vi "Updater Install Company Logo.vi"(8 "error in (no error)":errorcluster, 10 "Load? (F)":bool, 11 "Path to File":path) -> (0 "error out":errorcluster)   [LabVIEW 2011]
uses:
  <vilib>/picture/picture.llb/imagedata.ctl
panel:
  in  "Image Data":T1={"image type"=0, "image depth"=24, "image"=array[128820 elements], "mask"=[], "colors"=[], "Rectangle"={"left"=0, "top"=0, "right"=380, "bottom"=113}}
  in  "Company Logo":picture
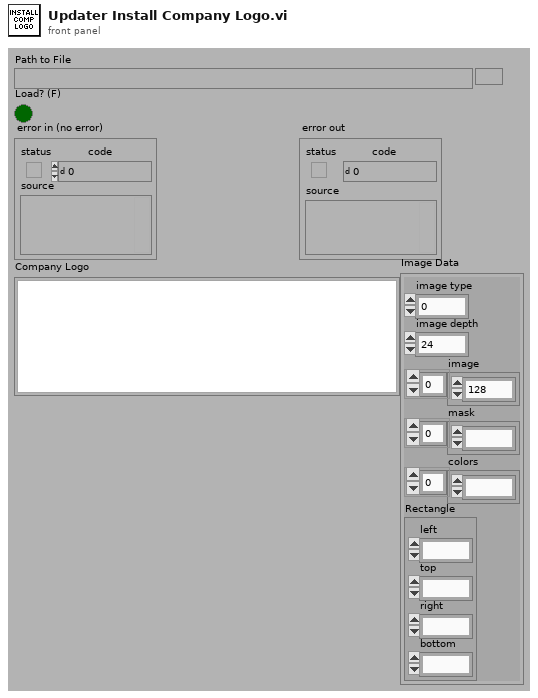
[diagram p1: front panel]
types:
  T1 = typedef "imagedata.ctl" = cluster{"image type":i32, "image depth":i32, "image":u8[], "mask":u8[], "colors":u32[], "Rectangle":cluster{"left":i16, "top":i16, "right":i16, "bottom":i16}}
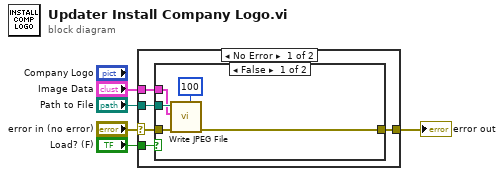
[diagram p0: block diagram]
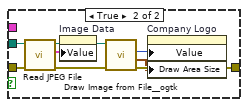
[diagram p2: hidden frame]
diagram:
  n1 = case shown="No Error" "error in (no error)" {
    selector: "error in (no error)" -> [w6 w24]
    tunnel: [w10 w24] -> w5
    tunnel: "Load? (F)" -> [w9 _]
    tunnel: "Path to File" -> [w8 _]
    tunnel: "Image Data" -> [w7 _]
    frame No Error {
      n2 = case shown="False" w9 {
        tunnel: w6 -> [w15 w20]
        tunnel: [w14 w23] -> w10
        tunnel: w8 -> [w12 w16]
        tunnel: w7 -> [w11 _]
        frame False {
          n3 = call <vilib>:"Write JPEG File.vi"("quality (80)"=100, "error in (no error)"=w15, "image data"=w11, "path to JPEG file"=w12) -> ("error out"=w14:errorcluster)  [unwired: 6 in, 1 out]
        }
        frame True {
          n4 = call <vilib>:"Read JPEG File.vi"("error in (no error)"=w20, "path to JPEG file"=w16) -> ("error out"=w19:errorcluster, "image data"=w18:T1, "path"=w17:path)  [unwired: 7 in]
          n5 = property on="Image Data" class="Clust (strict)"("Value"=w18) -> ()  [unwired: 2 in, 2 out]
          n6 = call "Draw Image from File__ogtk.vi"("error in (no error)"=w19, "path to image file"=w17) -> ("error out"=w23:errorcluster, "image size (pixels)"=w22:cluster{"x":i16, "y":i16}, "new picture"=w21:picture)  [unwired: 6 in, 1 out]
          n7 = property on="Company Logo" class="Pict"("Value"=w21, "Draw Area Size"=w22) -> ()  [unwired: 2 in, 2 out]
        }
      }
    }
    frame Error {
    }
  }
  "error out" <- w5
